vi "pre_filter_image.vi"(6 "Temp Image":T1, 7 "Gaussian Filter Size":dbl, 8 "error in (no error)":errorcluster, 9 "Mean Filter Size":i32, 10 "Output Image In":T1, 11 "Input Image":T1) -> (0 "error out":errorcluster, 3 "Output Image Out":T1)   [LabVIEW 2016]
uses:
  <vilib>/vision/Image Controls.llb/IMAQ Image.ctl
  <vilib>/vision/NI_Vision_Development_Module.lvlib
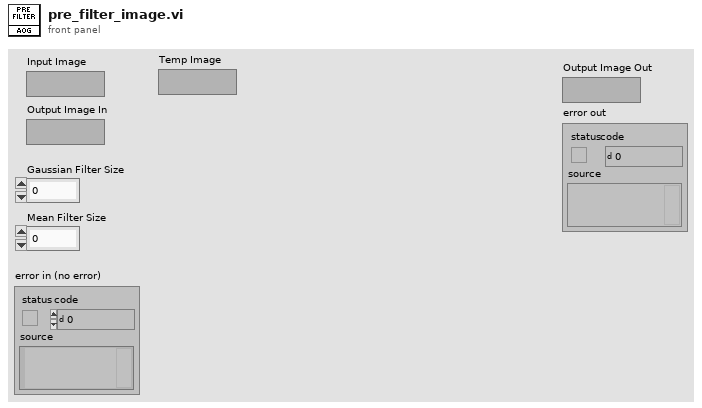
[diagram p1: front panel]
types:
  T1 = typedef "IMAQ Image.ctl" = refnum<image>
  T2 = typedef "Image Type" = u32
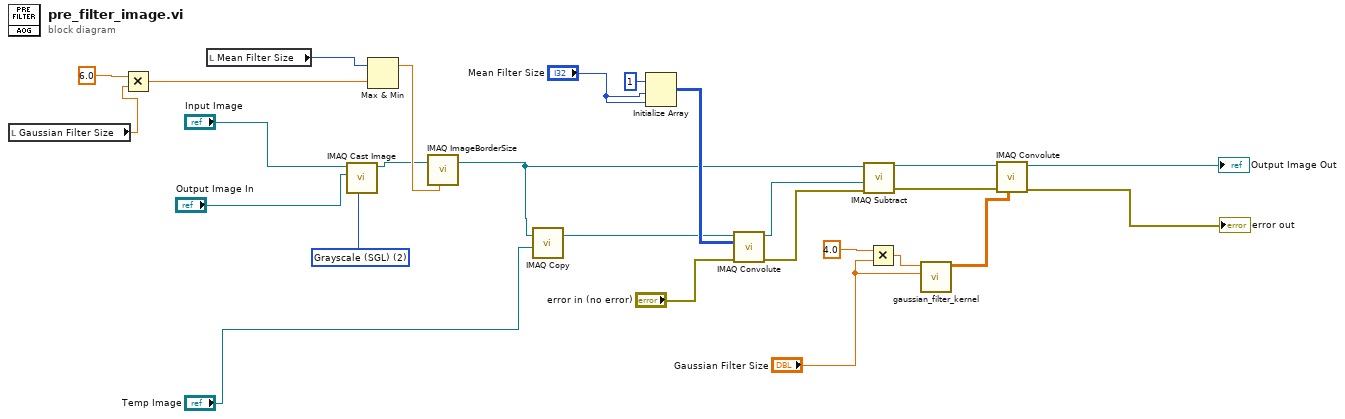
[diagram p0: block diagram]
diagram:
  w4 = T2 2 items=["Grayscale (U8)", "Grayscale (I16)", "Grayscale (SGL)", "Complex (CSG)", "RGB (U32)", "HSL (U32)", "RGB (U64)", "Grayscale (U16)"] ("Image Type")
  n1 = local read "Gaussian Filter Size"() -> (w6:dbl)
  n2 = Multiply(x=6.0, y=w6) -> (x*y=w7:dbl)
  n3 = local read "Mean Filter Size"() -> (w10:i32)
  n4 = call "IMAQ Cast Image"("Image Type"=w4, "Image Dst"="Output Image In", "Image Src"="Input Image") -> ("Image Dst Out"=w5:T1)  [unwired: 7 in, 1 out]
  n5 = Max & Min(x=w10, y=w7) -> (max(x,y)=w9:dbl)  [unwired: 1 out]
  n6 = call "IMAQ ImageBorderSize"("Image"=w5, "Image border size in"=w9) -> ("Image Out"=w11:T1)  [unwired: 2 in, 2 out]
  n7 = call "IMAQ Copy"("Image Dst"="Temp Image", "Image Src"=w11) -> ("Image Dst Out"=w24:T1)  [unwired: 4 in, 1 out]
  n8 = Initialize Array(u8 1 ("element"), "Mean Filter Size", "Mean Filter Size") -> (w25:u8[][])
  n9 = call "IMAQ Convolute"("Kernel"=w25, "error in (no error)"="error in (no error)", "Image Src"=w24) -> ("error out"=w15:errorcluster, "Image Dst Out"=w22:T1)  [unwired: 7 in]
  n10 = call "IMAQ Subtract"("Image Src A"=w11, "Image Src B"=w22, "error in (no error)"=w15) -> ("Image Dst Out"=w20:T1, "error out"=w14:errorcluster)  [unwired: 4 in]
  n11 = Multiply(x=4.0, y="Gaussian Filter Size") -> (x*y=w19:dbl)
  n12 = call "gaussian_filter_kernel.vi"("sigma"="Gaussian Filter Size", "size"=w19) -> ("Gaussian"=w21:dbl[][])  [unwired: 9 in]
  n13 = call "IMAQ Convolute"("Kernel"=w21, "error in (no error)"=w14, "Image Src"=w20) -> ("error out"=→"error out":errorcluster, "Image Dst Out"=→"Output Image Out":T1)  [unwired: 7 in]
